vi "rwfm_AcqRead(Wfm).vi"(6 "Timeout (s)":dbl=5.0, 7 "Poll Time (ms)":u32=10, 8 "error in":errorcluster, 9 "Samps Read per Chan":i32, 10 "Sampling Info":T2={"Number of Channels"=4, "Sampling Rate"=5120.0, "Channels"=[], "Units"=[], "Offsets"=[]}, 11 "Dynamic FPGA VI Reference":T1) -> (0 "error out":errorcluster, 1 "Samples Remaining":u32, 2 "Wfm Data":waveform(sgl)[](array[waveform]), 3 "Dynamic FPGA VI Reference":T1, 4 "Data Rate [S/s]":u32, 5 "Time Stamp":timestamp)   [LabVIEW 2017, in "cRIOWfmLibMcsa.lvlib"]
doc: "Reads waveform data from the DMA FIFO."
uses:
  <vilib>/addons/InsightCM/Devices/Shared/Mcsa/cRIOWfmAcqMcsa/cRIOWfmLibMcsa.lvlib
  <vilib>/addons/InsightCM/Devices/Shared/Cms/cRIOWfmAcq/subVIs/RIO Wfm Cust Ctrls/rwfm_SamplingInfo.ctl
  <vilib>/addons/InsightCM/Devices/Shared/Mcsa/cRIOWfmAcqMcsa/controls/rwfm_DynamicFPGArefMCSA.ctl
  <vilib>/Utility/error.llb/Error Cluster From Error Code.vi
  <vilib>/rvi/errors/niLvFpgaAdjustHostInterfaceError.vi
  <vilib>/rvi/interface/nirviReadWriteControl/nirviReadWriteControl.xnode
  <vilib>/rvi/interface/nirviMethod/nirviMethod.xnode
  NiFpgaLv.dll
  <vilib>/rvi/interface/Simulation/niFpgaSimulationCallBeginRW.vi
  <vilib>/FPGAPlugInAG/Dynamic/niLvFpga_ReadFifo_Dynamic.vi
  <vilib>/rvi/errors/niLvFpgaMergeErrorWithErrorCode.vi
  <vilib>/addons/InsightCM/Devices/Shared/Cms/cRIOWfmAcq/cRIOWfmLib.lvlib
panel:
  out "Read Time (ms)":u32
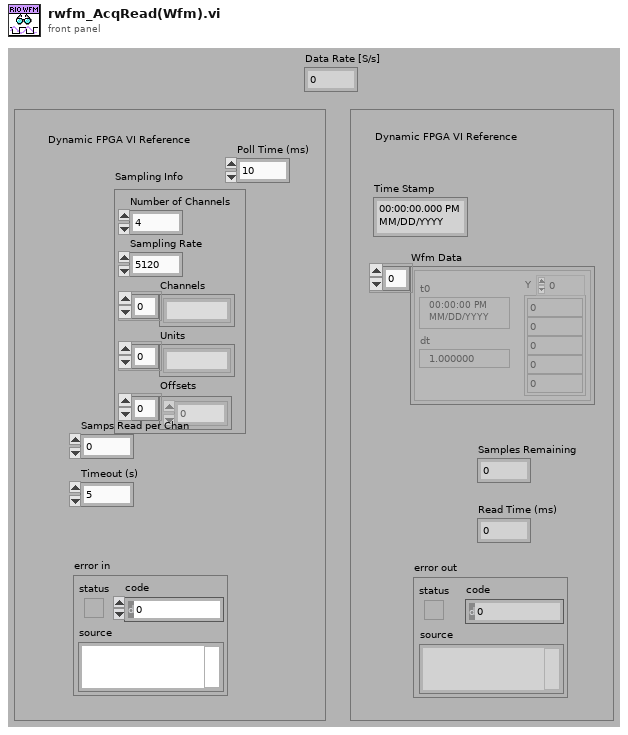
[diagram p1: front panel]
types:
  T1 = typedef "cRIOWfmLibMcsa.lvlib/rwfm_DynamicFPGArefMCSA.ctl" = refnum<k20>
  T2 = typedef "cRIOWfmLib.lvlib/rwfm_SamplingInfo.ctl" = cluster{"Number of Channels":i32, "Sampling Rate":dbl, "Channels":string[], "Units":string[], "Offsets":sgl[]}
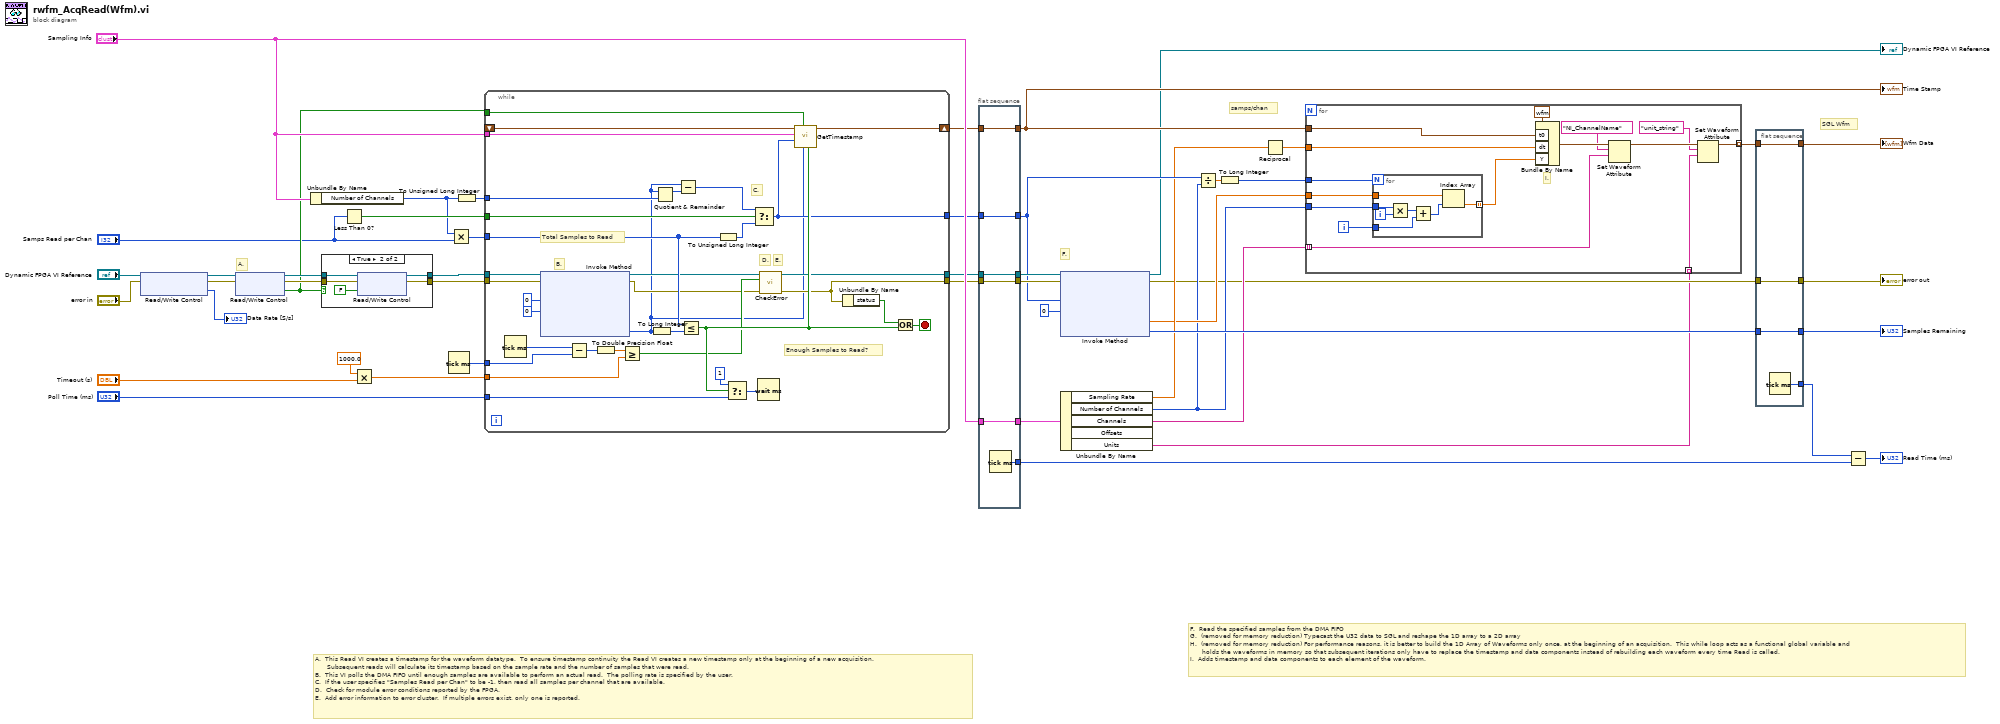
[diagram p0: block diagram]
diagram:
  # "samps/chan"
  # "SGL Wfm"
  # "F."
  # "F.  Read the specified samples from the DMA FIFO\nG.  (removed for memory reduction) Typecast the U32 data to SGL and reshape the 1D array to a 2D array\nH.  (removed for memory reduction) For performance reasons, it is better to build the 1D Array of Waveforms only once, at the beginning of an acquisition.  This while loop acts as a functional global variable and\n      holds the waveforms in memory so that subsequent iterations only have to replace the timestamp and data components instead of rebuilding each waveform every time Read is called.\nI.  Adds timestamp and data components to each element of the waveform."
  # "A.  This Read VI creates a timestamp for the waveform datatype.  To ensure timestamp continuity the Read VI creates a new timestamp only at the beginning of a new acquisition.  \n      Subsequent reads will calculate its timestamp based on the sample rate and the number of samples that were read.\nB.  This VI polls the DMA FIFO until enough samples are available to perform an actual read.  The polling rate is specified by the user.\nC.  If the user specifies \"Samples Read per Chan\" to be -1, then read all samples per channel that are available.\nD.  Check for module error conditions reported by the FPGA.\nE.  Add error information to error cluster.  If multiple errors exist, only one is reported."
  # "A."
  n1 = xnode "Read/Write Control"("FPGA VI Reference In"="Dynamic FPGA VI Reference", "error in"="error in") -> ("FPGA VI Reference Out"=w10:T1, "error out"=w13:errorcluster, "Data Rate [S/s]"=→"Data Rate [S/s]":u32)
  n2 = xnode "Read/Write Control"("FPGA VI Reference In"=w10, "error in"=w13) -> ("FPGA VI Reference Out"=w48:T1, "error out"=w49:errorcluster, "First Read"=w22:bool)
  n3 = Unbundle By Name("Sampling Info") -> ("Number of Channels"=w16:i32)
  n4 = case shown="True" w22 {
    tunnel: w48 -> [w51 w56]
    tunnel: [w51 w55] -> w47
    tunnel: w49 -> [w50 w54]
    tunnel: [w50 w53] -> w46
    frame False {
    }
    frame True {
      n5 = xnode "Read/Write Control"("FPGA VI Reference In"=w56, "error in"=w54, "First Read"=FALSE) -> ("FPGA VI Reference Out"=w55:T1, "error out"=w53:errorcluster)
    }
  }
  n6 = Less Than 0?(x="Samps Read per Chan") -> (x < 0?=w30:bool)
  n7 = Multiply(x=1000.0 ("y"), y="Timeout (s)") -> (x*y=w42:dbl)
  n8 = Tick Count (ms)() -> (millisecond timer value=w45:u32)
  n9 = Multiply(x=w16, y="Samps Read per Chan") -> (x*y=w29:i32)
  n10 = To Unsigned Long Integer(number=w16) -> (unsigned 32bit integer=w27:u32)
  n11 = while {
    tunnel: [w60] -> w33
    tunnel: [w63] -> w34
    tunnel: w22 -> [w79]
    tunnel: w47 -> [w83]
    tunnel: w46 -> [w82]
    shift-right: [w73] -> w32
    shift-left: _ -> [w80]
    tunnel: "Sampling Info" -> [w81]
    tunnel: w45 -> [w84]
    tunnel: w42 -> [w85]
    tunnel: "Poll Time (ms)" -> [w75]
    tunnel: w29 -> [w68]
    tunnel: [w66] -> w31
    tunnel: w30 -> [w71]
    tunnel: w27 -> [w67]
    stop <- w86 stop-if-true
    # "E."
    # "D."
    # "C."
    # "B."
    # "Total Samples to Read"
    # "Enough Samples to Read?"
    n12 = Tick Count (ms)() -> (millisecond timer value=w78:u32)
    n13 = xnode "Invoke Method"("FPGA VI Reference In"=w83, "error in"=w82, "Number of Elements"=u32 0, "Timeout (ms)"=0) -> ("FPGA VI Reference Out"=w62:T1, "error out"=w61:errorcluster, "Elements Remaining"=w57:u32)  [unwired: 1 out]
    n14 = Subtract(x=w78, y=w84) -> (x-y=w89:u32)
    n15 = To Double Precision Float(number=w89) -> (double precision float=w88:dbl)
    n16 = Greater Or Equal?(x=w88, y=w85) -> (x >= y?=w72:bool)
    n17 = To Long Integer(number=w57) -> (32bit integer=w70:i32)
    n18 = Quotient & Remainder(x=w57, y=w67) -> (x-y*floor(x/y)=w65:u32)  [unwired: 1 out]
    n19 = Subtract(x=w57, y=w65) -> (x-y=w64:u32)
    n20 = Less Or Equal?(x=w68, y=w70) -> (x <= y?=w77:bool)
    n21 = To Unsigned Long Integer(number=w68) -> (unsigned 32bit integer=w69:u32)
    n22 = Select(t=u32 1, s=w77, f=w75) -> (s? t:f=w76:u32)
    n23 = Select(t=w64, s=w71, f=w69) -> (s? t:f=w66:u32)
    n24 = Wait (ms)(milliseconds to wait=w76) -> ()  [unwired: 1 out]
    n25 = call <vilib>:"CheckError.vi"("error in (no error)"=w61, "timeout?"=w72, "dynamic fgpa vi reference in"=w62) -> ("error out"=w60:errorcluster, "dynamic fpga vi reference out"=w63:T1)  [unwired: 7 in]
    n26 = call <vilib>:"GetTimestamp.vi"("Enough Samples to Read"=w77, "Elements Remaining"=w57, "First Read"=w79, "Samples to Read"=w66, "Sampling Info"=w81, "Time Stamp in"=w80) -> ("Time Stamp out"=w73:timestamp)  [unwired: 5 in]
    n27 = Unbundle By Name(w60) -> ("status"=w87:bool)
    n28 = Or(x=w87, y=w77) -> (x .or. y?=w86:bool)
  }
  n29 = flat-sequence {
    tunnel: [w95] -> w14
    tunnel: "Sampling Info" -> [w94]
    tunnel: [w94] -> w36
    tunnel: [w93] -> w24
    tunnel: w34 -> [w93]
    tunnel: [w92] -> w23
    tunnel: w33 -> [w92]
    tunnel: [w91] -> w18
    tunnel: w32 -> [w91]
    tunnel: [w90] -> w21
    tunnel: w31 -> [w90]
    frame #0 {
      n30 = Tick Count (ms)() -> (millisecond timer value=w95:u32)
    }
  }
  n31 = xnode "Invoke Method"("FPGA VI Reference In"=w24, "error in"=w23, "Number of Elements"=w21, "Timeout (ms)"=0) -> ("FPGA VI Reference Out"=→"Dynamic FPGA VI Reference":T1, "error out"=w2:errorcluster, "Data"=w5:sgl[], "Elements Remaining"=w19:u32)
  n32 = Unbundle By Name(w36) -> ("Sampling Rate"=w7:dbl, "Number of Channels"=w4:i32, "Channels"=w8:string[], "Units"=w1:string[])  [unwired: 1 out]
  n33 = Divide(x=w21, y=w4) -> (x/y=w26:dbl)
  n34 = To Long Integer(number=w26) -> (32bit integer=w3:i32)
  n35 = Reciprocal(x=w7) -> (1/x=w6:dbl)
  n36 = for {
    tunnel: w18 -> [w101]
    tunnel: [w99] -> w25 mode=indexing
    tunnel: w8 -> [w109] mode=indexing
    tunnel: w6 -> [w102]
    tunnel: w5 -> [w106]
    tunnel: w4 -> [w105]
    tunnel: w3 -> [w103]
    tunnel: w1 -> [w97] mode=indexing
    i -> [w104]
    # "I."
    n37 = for {
      N: w103 -> [_]
      tunnel: w106 -> [w117]
      tunnel: w105 -> [w115]
      tunnel: w104 -> [w113]
      tunnel: [w111] -> w96 mode=indexing
      i -> [w116]
      n38 = Multiply(x=w115, y=w116) -> (x*y=w114:i32)
      n39 = Add(x=w114, y=w113) -> (x+y=w112:i32)
      n40 = Index Array(array=w117, index=w112) -> (element=w111:sgl)
    }
    n41 = Bundle By Name(cluster=waveform(sgl) {"t0"=timestamp(0 s since 1904-01-01), "dt"=1.0, "Y"=[]} ("waveform"), "t0"=w101, "dt"=w102, "Y"=w96) -> (w110:waveform(sgl))
    n42 = Set Waveform Attribute(5:w109, 6:"NI_ChannelName" ("name"), 7:w110) -> (3:w100:waveform(sgl))  [unwired: 1 in, 2 out]
    n43 = Set Waveform Attribute(5:w97, 6:"unit_string" ("name"), 7:w100) -> (3:w99:waveform(sgl))  [unwired: 1 in, 2 out]
  }
  n44 = flat-sequence {
    tunnel: [w121] -> w40
    tunnel: w2 -> [w121]
    tunnel: [w120] -> w37
    tunnel: w25 -> [w120]
    tunnel: [w119] -> w39
    tunnel: [w118] -> w28
    tunnel: w19 -> [w118]
    frame #0 {
      n45 = Tick Count (ms)() -> (millisecond timer value=w119:u32)
    }
  }
  n46 = Subtract(x=w39, y=w14) -> (x-y=→"Read Time (ms)":u32)
  "error out" <- w40
  "Samples Remaining" <- w28
  "Wfm Data" <- w37
  "Time Stamp" <- w18
